vi "FRCts20_Backend_ScriptCasesExample.vi"(8 "error in (no error)":errorcluster, 9 "Competition Start Date":timestamp, 11 "Path to Stats":path=path "C:/FRC Team Service/source/VI Source/FRCts20_Backend_GenerateStats.vi") -> (0 "error out":errorcluster)   [LabVIEW 2013, in "FRCts20_Backend_TestCode.lvlib"]
uses:
  FRCts20_Backend_TestCode.lvlib
  <vilib>/Utility/traverseref.llb/VI Scripting - Traverse.lvlib
  <vilib>/Utility/traverseref.llb/TRef TravTarget.ctl
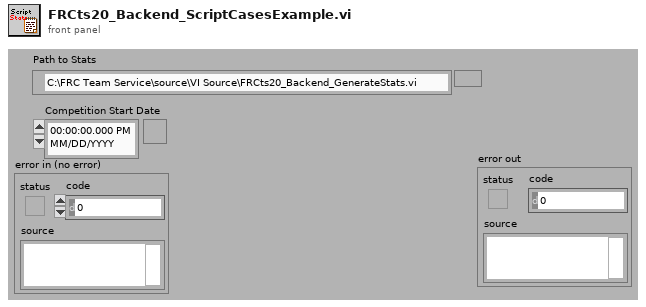
[diagram p1: front panel]
types:
  T1 = typedef "TRef TravTarget.ctl" = enum16{"FP", "BD", "Other"}
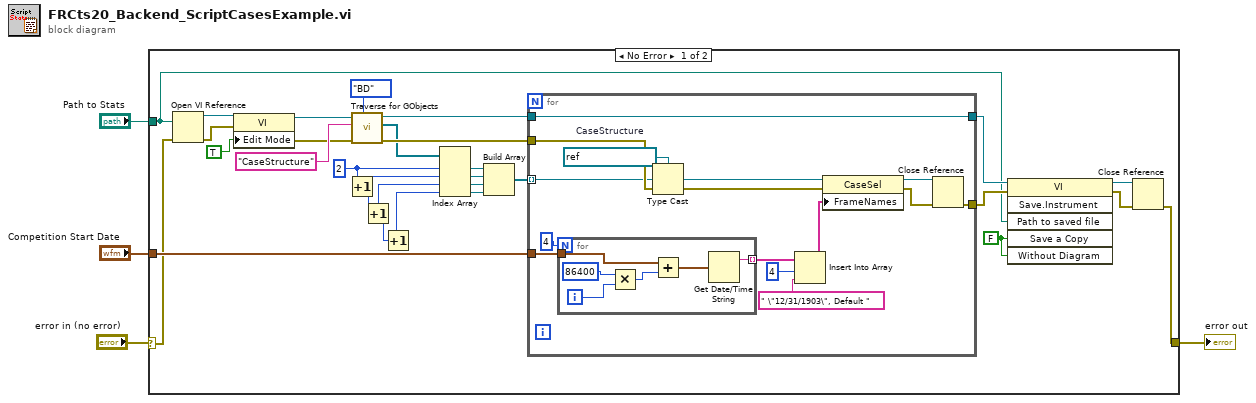
[diagram p0: block diagram]
diagram:
  n1 = case shown="No Error" "error in (no error)" {
    selector: "error in (no error)" -> [w6 w53]
    tunnel: "Competition Start Date" -> [w19 _]
    tunnel: "Path to Stats" -> [w9 _]
    tunnel: [w5 w53] -> w1
    frame No Error {
      w11 = FALSE ("Save a Copy")
      w24 = 2 ("index")
      n2 = Open VI Reference(vi path=w9, error in (no error)=w6) -> (vi reference=w17:refnum<vi>, error out=w15:errorcluster)  [unwired: 4 in]
      n3 = property class="VI"(reference=w17, error in=w15, "Edit Mode"=TRUE ("Edit Mode On Open")) -> (reference out=w13:refnum<vi>, error out=w14:errorcluster)
      n4 = Increment(x=w24) -> (x+1=w23:i32)
      n5 = call <vilib>:"Traverse for GObjects.vi"("Traverse Target"=TRef_TravTarget."BD", "error in (no error)"=w14, "Class Name"="CaseStructure", "VI Refnum"=w13) -> ("error out"=w30:errorcluster, "References"=w29:refnum<vi>[], "dup VI Refnum"=w18:refnum<vi>)  [unwired: 4 in, 1 out]
      n6 = Increment(x=w23) -> (x+1=w22:i32)
      n7 = Increment(x=w22) -> (x+1=w21:i32)
      n8 = Index Array(array=w29, index #1=w24, index #2=w23, index #3=w22, index #4=w21) -> (element #1=w28:refnum<vi>, element #2=w27:refnum<vi>, element #3=w26:refnum<vi>, element #4=w25:refnum<vi>)
      n9 = Build Array(w28, w27, w26, w25) -> (w20:refnum<vi>[])
      n10 = for {
        tunnel: w30 -> [w45]
        tunnel: w20 -> [w44] mode=indexing
        tunnel: w19 -> [w42]
        tunnel: [w38] -> w10
        tunnel: w18 -> [w37]
        tunnel: [w37] -> w12
        w46 = refnum<vi> refnum  # CaseStructure
        n11 = for {
          N: 4 -> [_]
          tunnel: w42 -> [w50]
          tunnel: [w47] -> w36 mode=indexing
          i -> [w48]
          n12 = Multiply(x=86400, y=w48) -> (x*y=w52:i32)
          n13 = Add(x=w50, y=w52) -> (x+y=w49:timestamp)
          n14 = Get Date/Time String(seconds (now)=w49) -> (date string=w47:string)  [unwired: 2 in, 1 out]
        }
        n15 = Type Cast(type=w46, x=w44) -> (*(type *) &x=w43:refnum<vi>)
        n16 = Insert Into Array(array=w36, index=4, new element=" \"12/31/1903\", Default " ("new element/subarray")) -> (w33:string[])
        n17 = property class="CaseSel"(reference=w43, error in=w45, "FrameNames"=w33) -> (reference out=w40:refnum<vi>, error out=w39:errorcluster)
        n18 = Close Reference(reference=w40, error in (no error)=w39) -> (error out=w38:errorcluster)
      }
      n19 = invoke class="VI" method="Save.Instrument"(reference=w12, error in=w10, "Path to saved file"=w9, "Save a Copy"=w11, "Without Diagram"=w11) -> (reference out=w8:refnum<vi>, error out=w7:errorcluster)  [unwired: 1 in, 4 out]
      n20 = Close Reference(reference=w8, error in (no error)=w7) -> (error out=w5:errorcluster)
    }
    frame Error {
    }
  }
  "error out" <- w1
